vi "Schedule Is Active.vi"(10 "iteration":u64=1, 11 "Schedule in":T1) -> (2 "active?":bool, 3 "Schedules out":T1)   [LabVIEW 2017, in "DSF Core.lvlib" / "Scheduler.lvclass"]
uses:
  Scheduler.lvclass
  Transfer Group Scheduler Data.ctl
  Timing/Timing.lvclass
  Timing/Timing.lvclass/Timing.ctl
  Timing/Get Decimation.vi
  Timing/Get Offset.vi
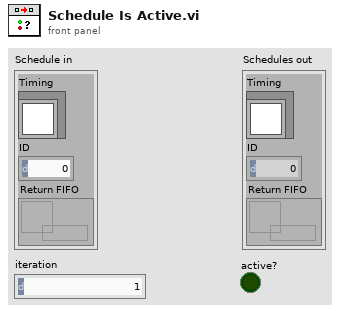
[diagram p1: front panel]
types:
  T1 = typedef "DSF Core.lvlib/Scheduler.lvclass/Transfer Group Scheduler Data.ctl" = cluster{"Timing":refnum<class "Timing.lvclass">, "ID":i32, "Return FIFO":refnum<k33>}
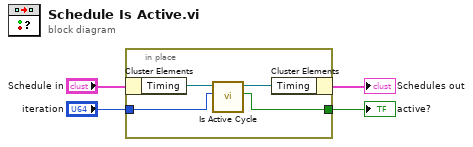
[diagram p0: block diagram]
diagram:
  n1 = in-place {
    in-place-border: "iteration" -> [w6]
    in-place-border: [w5] -> w1
    n2 = in-place-cluster #1("Schedule in") -> ("Timing"=w8:refnum<class "Timing.lvclass">)
    n3 = call "Is Active Cycle.vi"("iteration"=w6, "Timing in"=w8) -> ("active?"=w5:bool, "Timing out"=w7:refnum<class "Timing.lvclass">)  [unwired: 8 in]
    n4 = in-place-cluster #1("Timing"=w7) -> (→"Schedules out":T1)
  }
  "active?" <- w1
